vi "shutter vi_MD.vi"() -> ()   [LabVIEW 2012]
uses:
  <vilib>/DAQmx/write.llb/DAQmx Write (Digital Bool 1Line 1Point).vi
  GFG/GFGstringGet.vi
  <vilib>/DAQmx/create/channels.llb/DAQmx Create Channel (DO-Digital Output).vi
  <vilib>/DAQmx/miscellaneous.llb/DAQmx Fill In Error Info.vi
  GFG/GFG library.lvlib
panel:
  in  "Clear":bool
  out "Source VI":string
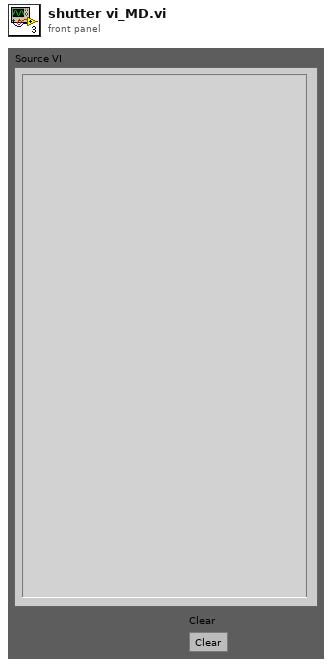
[diagram p1: front panel]
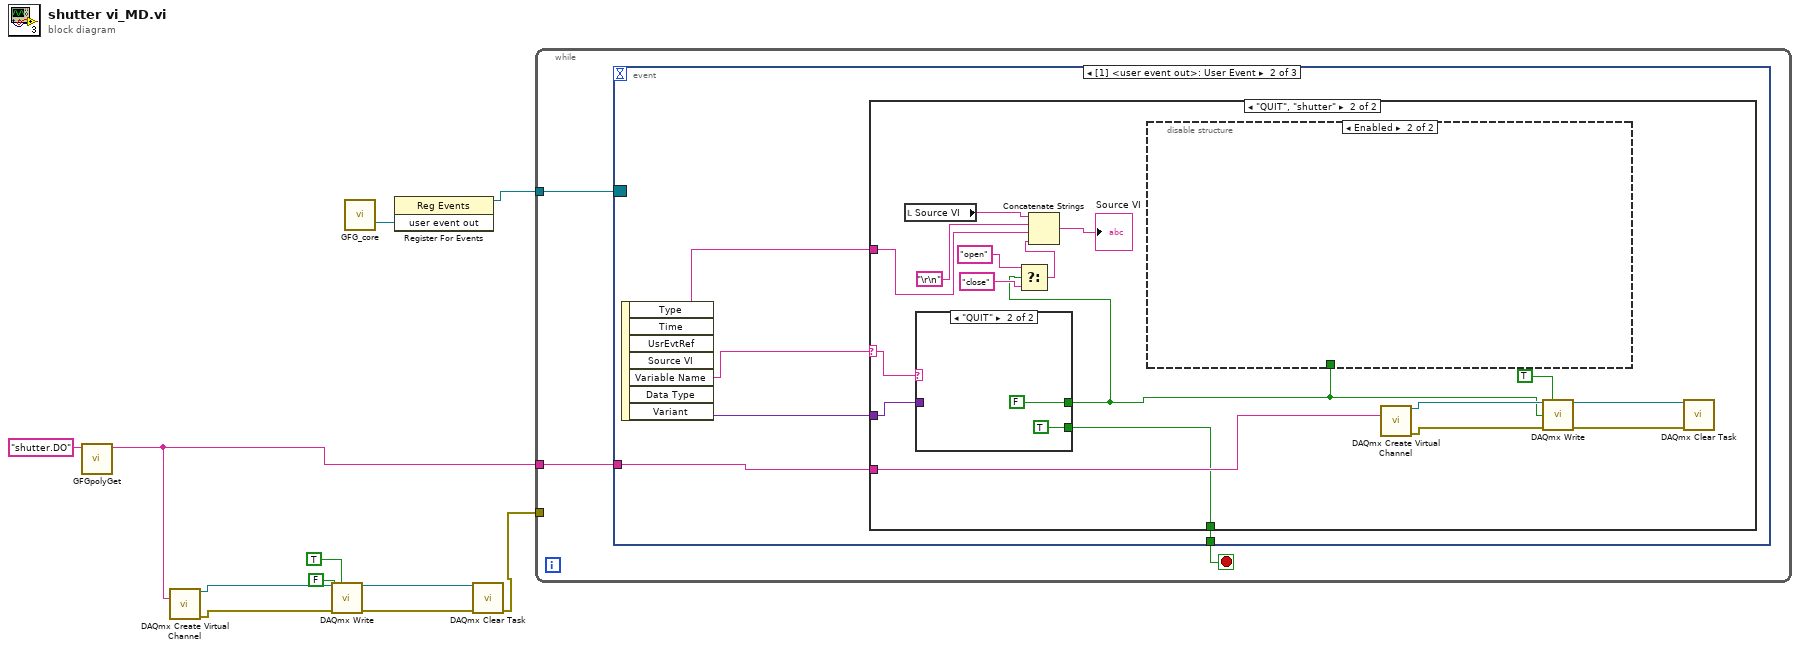
[diagram p0: block diagram]
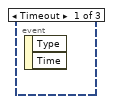
[diagram p2: hidden frame]
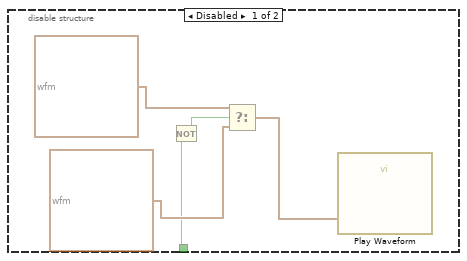
[diagram p4: hidden frame]
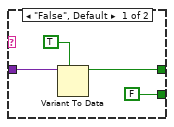
[diagram p5: hidden frame]
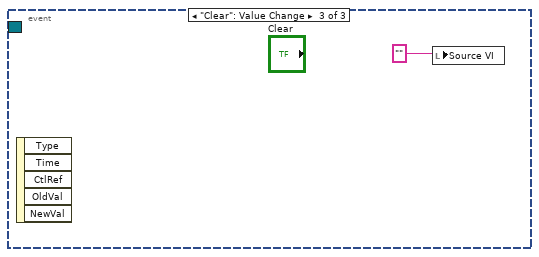
[diagram p6: hidden frame]
diagram:
  n1 = call-poly "GFGpolyGet.vi"("Variable Name in"="shutter.DO" ("Tag in")) -> ("String"=w3:string)  [unwired: 10 in]
  n2 = call-poly <vilib>:"DAQmx Create Virtual Channel.vi"("lines"=w3) -> ("task out"=w4:refnum<k21>, "error out"=w8:errorcluster)  [unwired: 13 in]
  n3 = call-poly <vilib>:"DAQmx Write.vi"("task/channels in"=w4, "auto start"=TRUE, "data"=FALSE, "error in"=w8) -> ("task out"=w6:refnum<k21>, "error out"=w7:errorcluster)  [unwired: 9 in, 1 out]
  n4 = call "GFG_core.vi"() -> ("user event out"=w11:refnum<user-event>)  [unwired: 13 in, 6 out]
  n5 = register-events(w11) -> (reference out=w10:refnum<event-registration>)  [unwired: 2 in, 1 out]
  n6 = call <vilib>:"DAQmx Clear Task.vi"("task in"=w6, "error in"=w7) -> ("error out"=w1:errorcluster)  [unwired: 13 in]
  n7 = while {
    tunnel: w10 -> [w14]
    tunnel: w3 -> [w12]
    tunnel: w1 -> [_]
    stop <- w13 stop-if-true
    n8 = event shown="[1] <user event out>: User Event" {
      selector: w14 -> [_ _ _]
      dyn-events: _ -> [_ _ _]
      timeout: _ -> [_ _ _]
      tunnel: [_ w16 _] -> w13
      tunnel: w12 -> [_ w17 _]
      event Timeout {
        n9 = event-data() -> ()  [unwired: 1 in, 2 out]
      }
      event User Event {
        n10 = event-data() -> ("Source VI"=w15:string, "Variable Name"=w19:string, "Variant"=w18:variant)  [unwired: 1 in, 4 out]
        n11 = case shown="\"QUIT\", \"shutter\"" w19 {
          selector: w19 -> [_ w29]
          tunnel: w18 -> [_ w36]
          tunnel: w17 -> [_ w35]
          tunnel: [_ w28] -> w16
          tunnel: w15 -> [_ w24]
          frame "False", Default {
          }
          frame "QUIT", "shutter" {
            n12 = local read "Source VI"() -> (w27:string)
            n13 = case shown="\"QUIT\"" w29 {
              tunnel: w36 -> [w45 _]
              tunnel: [w43 FALSE] -> w21
              tunnel: [FALSE TRUE] -> w28
              frame "False", Default {
                n14 = Variant To Data(type=TRUE, Variant=w45) -> (data=w43:bool)  [unwired: 1 in, 1 out]
              }
              frame "QUIT" {
              }
            }
            n15 = Select(t="open" ("Source VI"), s=w21, f="close" ("Source VI")) -> (s? t:f=w20:string)
            n16 = Concatenate Strings(w27, "\r\n", w24, w20) -> (→"Source VI":string)
            n17 = disable-structure shown="Enabled" {
              disable-tunnel: w21 -> [w38 _]
              frame Disabled {
                n18 = Not(x=w38) -> (.not. x?=w37:bool)
                n19 = Select(t=waveform(dbl) {"t0"=timestamp(0 s since 1904-01-01), "dt"=9.070294784580499e-05, "Y"=array[2000 elements]} ("output waveform"), s=w37, f=waveform(dbl) {"t0"=timestamp(0 s since 1904-01-01), "dt"=4.5351473922902495e-05, "Y"=array[1700 elements]} ("output waveform")) -> (s? t:f=w39:waveform(dbl))
                n20 = call "Play Waveform"("Data"=w39) -> ()  [unwired: 18 in, 1 out]
              }
              frame Enabled {
              }
            }
            n21 = call-poly <vilib>:"DAQmx Create Virtual Channel.vi"("lines"=w35) -> ("task out"=w34:refnum<k21>, "error out"=w30:errorcluster)  [unwired: 13 in]
            n22 = call-poly <vilib>:"DAQmx Write.vi"("task/channels in"=w34, "auto start"=TRUE, "data"=w21, "error in"=w30) -> ("task out"=w32:refnum<k21>, "error out"=w31:errorcluster)  [unwired: 9 in, 1 out]
            n23 = call <vilib>:"DAQmx Clear Task.vi"("task in"=w32, "error in"=w31) -> ()  [unwired: 13 in, 1 out]
          }
        }
      }
      event "Clear": Value Change {
        n24 = event-data() -> ()  [unwired: 1 in, 5 out]
        n25 = local write "Source VI"("" ("Source VI")) -> ()
      }
    }
  }
